vi "GetLoopConditional.vi"(6 "error in":errorcluster, 9 "ForLoop in":refnum<class "ForLoop.lvclass">) -> (0 "error out":errorcluster, 3 "ForLoop out":refnum<class "ForLoop.lvclass">, 4 "conditional UID":i32)   [LabVIEW 2014, in "Raspberry Pi Compatible Compiler for LabVIEW.lvlib" / "ForLoop.lvclass"]
uses:
  ForLoop.lvclass
  ForLoop.lvclass/ForLoop.ctl
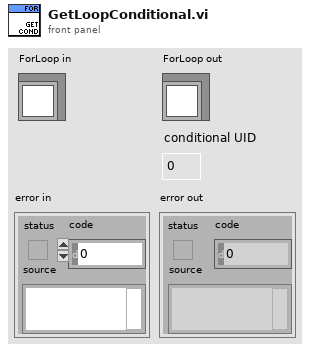
[diagram p1: front panel]
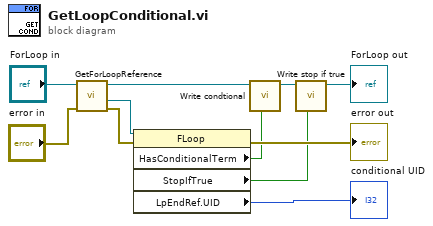
[diagram p0: block diagram]
diagram:
  n1 = call "GetForLoopReference.vi"("error in"="error in", "ForLoop in"="ForLoop in") -> ("error out"=w8:errorcluster, "reference out"=w9:refnum<vi>, "ForLoop out"=w5:refnum<class "ForLoop.lvclass">)  [unwired: 7 in]
  n2 = property class="FLoop"(reference=w9, error in=w8) -> (error out=→"error out":errorcluster, "HasConditionalTerm"=w6:bool, "StopIfTrue"=w4:bool, "LpEndRef.UID"=→"conditional UID":i32)  [unwired: 1 out]
  n3 = call "Write condtional.vi"("condtional"=w6, "ForLoop in"=w5) -> ("ForLoop out"=w1:refnum<class "ForLoop.lvclass">)  [unwired: 7 in]
  n4 = call "Write stop if true.vi"("stop if true"=w4, "ForLoop in"=w1) -> ("ForLoop out"=→"ForLoop out":refnum<class "ForLoop.lvclass">)  [unwired: 7 in]
